vi "Z6_Beamline.set Status Subscriber Information.vi"(0 "i ref in":refnum<vi>, 5 "error in (no error)":errorcluster) -> (14 "i ref out":refnum<vi>, 19 "error out":errorcluster)   [LabVIEW 2014, in "Z6_Beamline.lvlib"]
doc: "This VI sets relevant Information for Status Subscriber."
uses:
  Z6_Beamline.lvlib
  PH_BL-Master/PH_BL-Master.Status Subscriber Information.ctl
  PH_BL-Master/PH_BL-Master.Attribute Set.ctl
  Z6_Beamline.Switch Instances.ctl
  Z6_Beamline.Black Box Instances.ctl
  PH_BL-Master/PH_BL-Master.lvlib
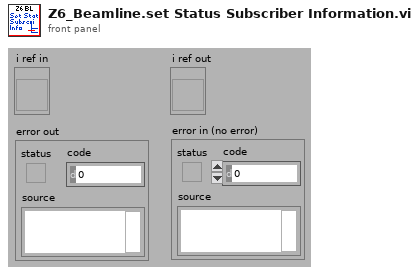
[diagram p1: front panel]
types:
  T1 = typedef "Z6_Beamline.lvlib/Z6_Beamline.i attribute.ctl" = cluster{"Subs ok GUI Refs":T2, "Refs BL Northtower":refnum<vi>[], "Refs BL Southtower":refnum<vi>[], "Refs BL 100TW COS":refnum<vi>[], "State Subsystems":cluster{"Northtower":bool, "Southtower":bool, "Frontends":bool, "100TW COS":bool}, "Z6 Beamline Status Subscriber Information":T3, "Color State PHELIX":i16}
  T2 = typedef "Z6_Beamline.lvlib/Z6_Beamline.Subsystem ok GUI Refs.ctl" = cluster{"Northtower ok":refnum<vi>, "Southtower ok":refnum<vi>, "Frontends ok":refnum<vi>, "100TW COS ok":refnum<vi>}
  T3 = typedef "Z6_Beamline.lvlib/Z6_Beamline.Status Subscriber Information.ctl" = cluster{"BL Z6 Shutter":T4, "CH 10":T4, "CH 11":T4, "ST Flip Cam":T4, "ST Flip DB":T4, "BL Z6 Dump":T4}
  T4 = typedef "PH_BL-Master.lvlib/PH_BL-Master.Status Subscriber Information.ctl" = cluster{"Index of element":i32, "Attributeset":T5}
  T5 = typedef "PH_BL-Master.lvlib/PH_BL-Master.Attribute Set.ctl" = enum16{"Boolean Status Service Subscriber", "Picture Status Service Subscriber"}
  T6 = typedef "Z6_Beamline.lvlib/Z6_Beamline.Switch Instances.ctl" = string
  T7 = typedef "Z6_Beamline.lvlib/Z6_Beamline.Black Box Instances.ctl" = string
  T8 = cluster{"[0]":T4, "[1]":T4, "[2]":T4, "[3]":T4, "[4]":T4, "[5]":T4}
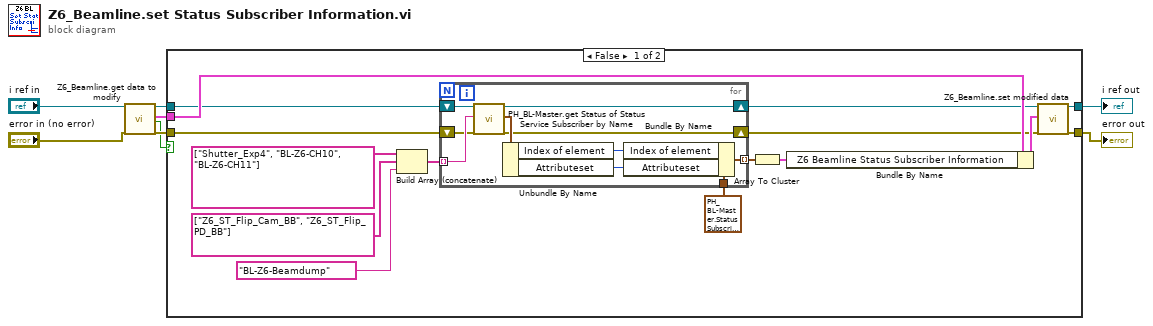
[diagram p0: block diagram]
diagram:
  n1 = call "Z6_Beamline.get data to modify.vi"("i ref in"="i ref in", "error in (no error)"="error in (no error)") -> ("i ref out"=w6:refnum<vi>, "i attribute"=w2:T1, "timed out"=w3:bool, "error out"=w4:errorcluster)  [unwired: 14 in]
  n2 = case shown="False" w3 {
    tunnel: w6 -> [w16 w35]
    tunnel: [w23 w35] -> w5
    tunnel: w4 -> [w14 w34]
    tunnel: w2 -> [w17 _]
    tunnel: [w21 w34] -> w1
    frame False {
      n3 = Build Array (concatenate)(T6[] ["Shutter_Exp4", "BL-Z6-CH10", "BL-Z6-CH11"], T7[] ["Z6_ST_Flip_Cam_BB", "Z6_ST_Flip_PD_BB"], T6 "BL-Z6-Beamdump" ("Z6 Switch Instances")) -> (w18:T6[])
      n4 = for {
        tunnel: T4 {"Index of element"=0, "Attributeset"=enum."Boolean Status Service Subscriber"} ("Status Subscriber Information.fs Exit Shutter") -> [w33]
        tunnel: [w32] -> w20 mode=indexing
        tunnel: w18 -> [w28] mode=indexing
        shift-right: [w25] -> w15
        shift-left: w16 -> [w27]
        shift-right: [w24] -> w13
        shift-left: w14 -> [w26]
        n5 = call "PH_BL-Master.get Status of Status Service Subscriber by Name.vi"("i ref in"=w27, "Status Subscriber Instance"=w28, "error in (no error)"=w26) -> ("i ref out"=w25:refnum<vi>, "Status Subscriber Information"=w31:T4, "error out"=w24:errorcluster)  [unwired: 14 in]
        n6 = Unbundle By Name(w31) -> ("Index of element"=w30:i32, "Attributeset"=w29:T5)
        n7 = Bundle By Name(cluster=w33, "Index of element"=w30, "Attributeset"=w29) -> (w32:T4)
      }
      n8 = Array To Cluster(array=w20) -> (cluster=w12:T8)
      n9 = Bundle By Name(cluster=w17, "Z6 Beamline Status Subscriber Information"=w12) -> (w22:T1)
      n10 = call "Z6_Beamline.set modified data.vi"("i ref in"=w15, "i attribute"=w22, "error in (no error)"=w13) -> ("i ref out"=w23:refnum<vi>, "error out"=w21:errorcluster)  [unwired: 15 in]
    }
    frame True {
    }
  }
  "i ref out" <- w5
  "error out" <- w1
